vi "GetDBPathPure.vi"(1 "Filename":string) -> (0 "Connection":path)   [LabVIEW 2014]
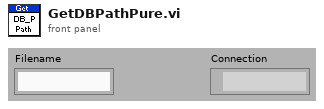
[diagram p1: front panel]
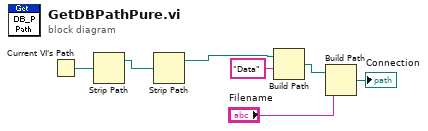
[diagram p0: block diagram]
diagram:
  n1 = Current VI's Path() -> (path=w4:path)
  n2 = Strip Path(path=w4) -> (stripped path=w3:path)  [unwired: 1 out]
  n3 = Strip Path(path=w3) -> (stripped path=w2:path)  [unwired: 1 out]
  n4 = Build Path(base path=w2, name or relative path="Data") -> (appended path=w7:path)
  n5 = Build Path(base path=w7, name or relative path="Filename") -> (appended path=→"Connection":path)
